vi "Replace Outside Typedef Ctrl.vi"(8 "error in":errorcluster, 10 "non-library vi[]":string[](array[string]), 11 "target directory":path) -> (0 "error out":errorcluster)   [LabVIEW 2021, in "Converter.lvlib"]
uses:
  Converter.lvlib
  Converter Reusables/Converter Reusables.lvlib
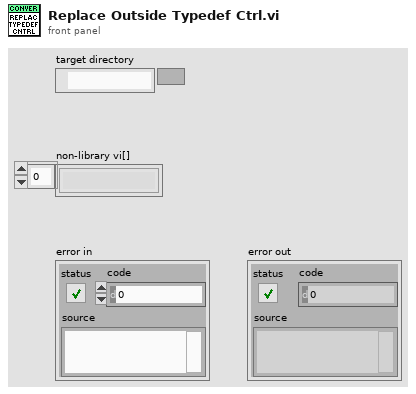
[diagram p1: front panel]
types:
  T1 = enum32{"not a typedef", "typedef", "strict typedef", "class private data"}
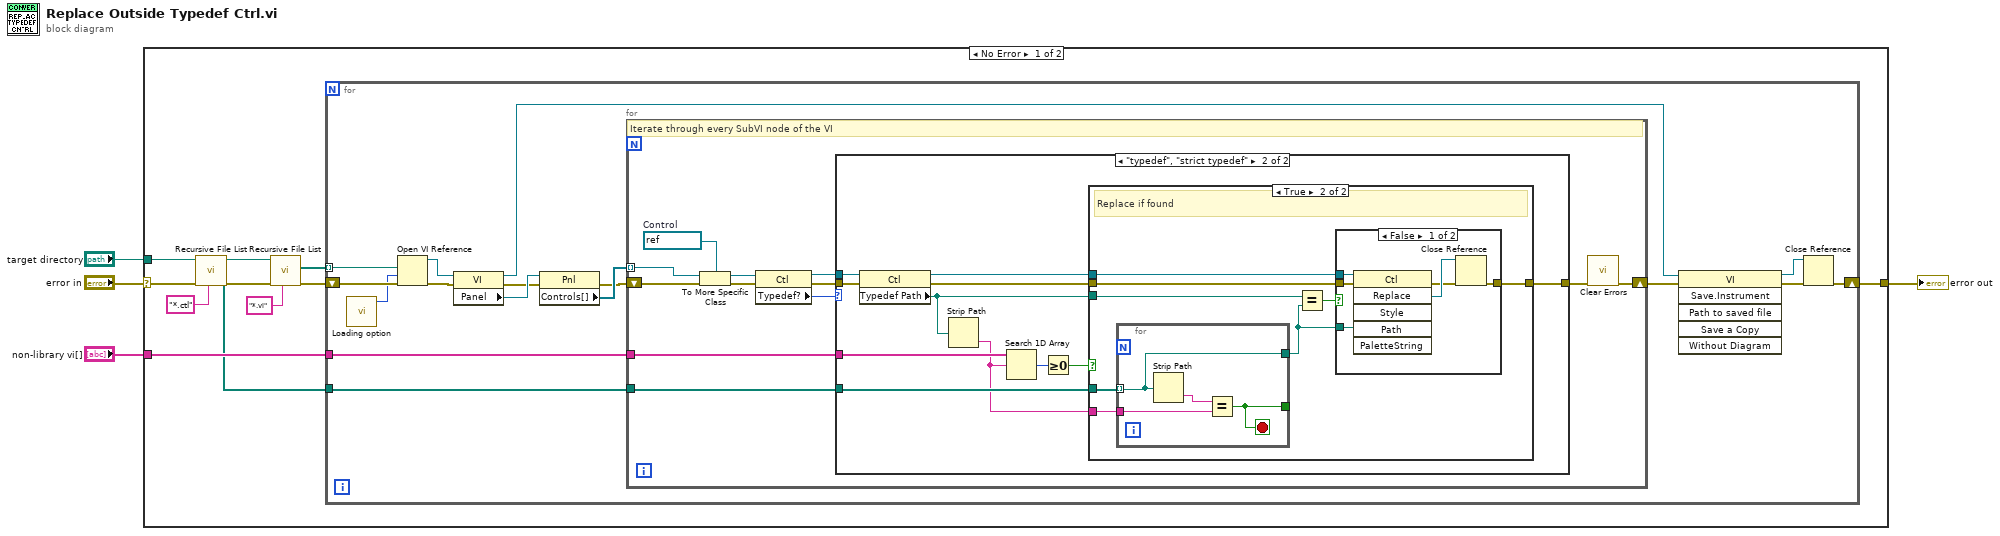
[diagram p0: block diagram]
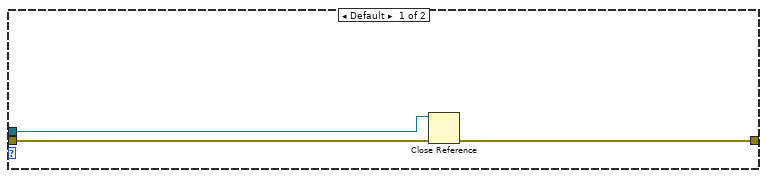
[diagram p2: hidden frame]
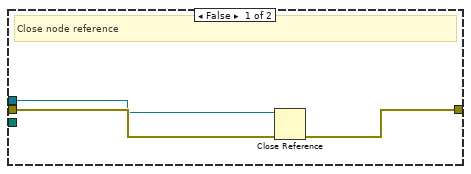
[diagram p3: hidden frame]
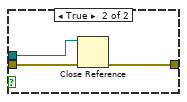
[diagram p4: hidden frame]
diagram:
  n1 = case shown="No Error" "error in" {
    selector: "error in" -> [w10 w82]
    tunnel: "non-library vi[]" -> [w15 _]
    tunnel: [w12 w82] -> w3
    tunnel: "target directory" -> [w8 _]
    frame No Error {
      n2 = call <vilib>:"Recursive File List.vi"("pattern"="*.ctl", "error in (no error)"=w10, "Folder Path"=w8) -> ("error out"=w9:errorcluster, "All Files in Dir"=w6:path[], "dup Folder Path"=w7:path)  [unwired: 4 in, 2 out]
      n3 = call <vilib>:"Recursive File List.vi"("pattern"="*.vi", "error in (no error)"=w9, "Folder Path"=w7) -> ("error out"=w14:errorcluster, "All Files in Dir"=w5:path[])  [unwired: 4 in, 3 out]
      n4 = for {
        tunnel: w6 -> [w30]
        tunnel: w15 -> [w29]
        tunnel: w5 -> [w23] mode=indexing
        shift-right: [w24] -> w12
        shift-left: w14 -> [w26]
        n5 = call "Loading option.vi"() -> ("options"=w18:i32)  [unwired: 11 in]
        n6 = Open VI Reference(vi path=w23, options=w18, error in (no error)=w26) -> (vi reference=w19:refnum<vi>, error out=w25:errorcluster)  [unwired: 3 in]
        n7 = property class="VI"(reference=w19, error in=w25) -> (reference out=w21:refnum<vi>, error out=w16:errorcluster, "Panel"=w17:refnum<vi>)
        n8 = property class="Pnl"(reference=w17, error in=w16) -> (error out=w28:errorcluster, "Controls[]"=w31:refnum<vi>[])  [unwired: 1 out]
        n9 = for {
          tunnel: w31 -> [w34] mode=indexing
          shift-right: [w32] -> w27
          shift-left: w28 -> [w43]
          tunnel: w29 -> [w36]
          tunnel: w30 -> [w40]
          w38 = refnum<vi> refnum  # Control
          # "Iterate through every SubVI node of the VI"
          n10 = To More Specific Class(target class=w38, reference=w34, error in=w43) -> (specific class reference=w39:refnum<vi>, error out=w37:errorcluster)
          n11 = property class="Ctl"(reference=w39, error in=w37) -> (reference out=w33:refnum<vi>, error out=w42:errorcluster, "Typedef?"=w35:T1)
          n12 = case shown="\"typedef\", \"strict typedef\"" w35 {
            tunnel: w42 -> [w46 w56]
            tunnel: w33 -> [w44 w50]
            tunnel: [w45 w55] -> w41
            tunnel: w40 -> [_ w53]
            tunnel: w36 -> [_ w52]
            frame Default {
              n13 = Close Reference(reference=w44, error in (no error)=w46) -> (error out=w45:errorcluster)
            }
            frame "typedef", "strict typedef" {
              n14 = property class="Ctl"(reference=w50, error in=w56) -> (reference out=w49:refnum<vi>, error out=w51:errorcluster, "Typedef Path"=w47:path)
              n15 = Strip Path(path=w47) -> (name=w48:string)  [unwired: 1 out]
              n16 = Search 1D Array(1D array=w52, element=w48) -> (index of element=w57:i32)  [unwired: 1 in]
              n17 = Greater Or Equal To 0?(x=w57) -> (x >= 0?=w54:bool)
              n18 = case shown="True" w54 {
                tunnel: w51 -> [w60 w68]
                tunnel: w49 -> [w59 w67]
                tunnel: [w58 w64] -> w55
                tunnel: w53 -> [_ w66]
                tunnel: w48 -> [_ w65]
                tunnel: w47 -> [_ w63]
                frame False {
                  # "Close node reference"
                  n19 = Close Reference(reference=w59, error in (no error)=w60) -> (error out=w58:errorcluster)
                }
                frame True {
                  # "Replace if found"
                  n20 = for {
                    tunnel: w66 -> [w79] mode=indexing
                    tunnel: w65 -> [w80]
                    tunnel: [w79] -> w62
                    tunnel: [w78] -> _
                    stop <- w78 stop-if-true
                    n21 = Strip Path(path=w79) -> (name=w81:string)  [unwired: 1 out]
                    n22 = Equal?(x=w81, y=w80) -> (x = y?=w78:bool)
                  }
                  n23 = Equal?(x=w63, y=w62) -> (x = y?=w61:bool)
                  n24 = case shown="False" w61 {
                    tunnel: w68 -> [w74 w77]
                    tunnel: w67 -> [w73 w75]
                    tunnel: [w70 w76] -> w64
                    tunnel: w62 -> [w69 _]
                    frame False {
                      n25 = invoke class="Ctl" method="Replace"(reference=w73, error in=w74, "Path"=w69) -> (error out=w71:errorcluster, "Replace"=w72:refnum<vi>)  [unwired: 3 in, 4 out]
                      n26 = Close Reference(reference=w72, error in (no error)=w71) -> (error out=w70:errorcluster)
                    }
                    frame True {
                      n27 = Close Reference(reference=w75, error in (no error)=w77) -> (error out=w76:errorcluster)
                    }
                  }
                }
              }
            }
          }
          n28 = call <vilib>:"Clear Errors.vi"("error in (no error)"=w41) -> ("error out"=w32:errorcluster)  [unwired: 5 in, 1 out]
        }
        n29 = invoke class="VI" method="Save.Instrument"(reference=w21, error in=w27) -> (reference out=w20:refnum<vi>, error out=w22:errorcluster)  [unwired: 4 in, 4 out]
        n30 = Close Reference(reference=w20, error in (no error)=w22) -> (error out=w24:errorcluster)
      }
    }
    frame Error {
    }
  }
  "error out" <- w3
